vi "Save Waveform to Reference Channel.vi"(8 "error in (no error)":errorcluster, 9 "Memory Location (0: Reference A)":i32(ring) items=["Reference A", "Reference B", "Reference C", "Reference D"], 10 "Channel (0: Channel 1)":i32(ring) items=["Channel 1", "Channel 2", "Channel 3", "Channel 4", "Math", "FFT"], 11 "VISA resource name":refnum<visa-resource-name>) -> (0 "error out":errorcluster, 3 "VISA resource name out":refnum<visa-resource-name>)   [LabVIEW 2015, in "Tektronix TDS 200 1000 2000 Series.lvlib"]
doc: "Saves a waveform to internal memory."
uses:
  <instrlib>/Tektronix TDS 200 1000 2000 Series/Tektronix TDS 200 1000 2000 Series.lvlib
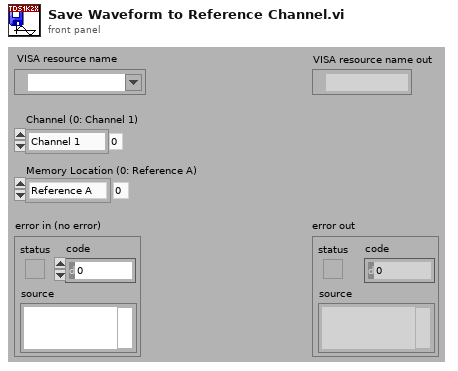
[diagram p1: front panel]
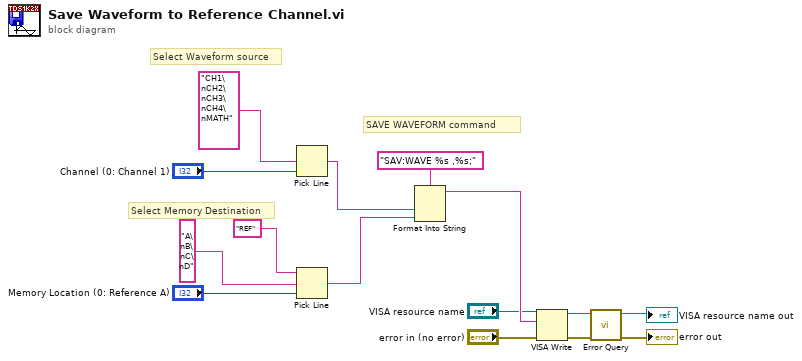
[diagram p0: block diagram]
diagram:
  # "Select Memory Destination"
  # "Select Waveform source"
  # "SAVE WAVEFORM command"
  n1 = Pick Line(multi-line string="CH1\nCH2\nCH3\nCH4\nMATH", line index="Channel (0: Channel 1)") -> (output string=w5:string)  [unwired: 1 out]
  n2 = Pick Line(string ("")="REF", multi-line string="A\nB\nC\nD", line index="Memory Location (0: Reference A)") -> (output string=w11:string)
  n3 = Format Into String(format string="SAV:WAVE %s ,%s;", w5, w11) -> (resulting string=w10:string)  [unwired: 2 in, 1 out]
  n4 = VISA Write(VISA resource name="VISA resource name", write buffer=w10, error in (no error)="error in (no error)") -> (VISA resource name out=w3:refnum<visa-resource-name>, error out=w4:errorcluster)  [unwired: 1 out]
  n5 = call <instrlib>:"Error Query.vi"("error in (no error)"=w4, "VISA resource name"=w3) -> ("error out"=→"error out":errorcluster, "VISA resource name out"=→"VISA resource name out":refnum<visa-resource-name>)  [unwired: 8 out]
